vi "createOuterLoopClockIRQ.vi"(8 "error in (no error)":errorcluster, 11 "Boot in":refnum<class "Boot.lvclass">) -> (0 "error out":errorcluster, 2 "OuterLoopClockIRQ":refnum<class "IIRQ.lvclass">, 3 "Boot out":refnum<class "Boot.lvclass">)   [LabVIEW 2016, in "Boot.lvclass"]
uses:
  Boot.lvclass
  Common_RT_FPGA/IIRQ/IIRQ.lvclass
  Resources/OuterLoopClockIRQ/OuterLoopClockIRQ.lvclass
  D:/Code/ts_M1M3Support/Common_RT_FPGA/IIRQ/IIRQ.lvclass
  Boot.lvclass/Boot.ctl
  Resources/OuterLoopClockIRQ/OuterLoopClockIRQ.lvclass/OuterLoopClockIRQ.ctl
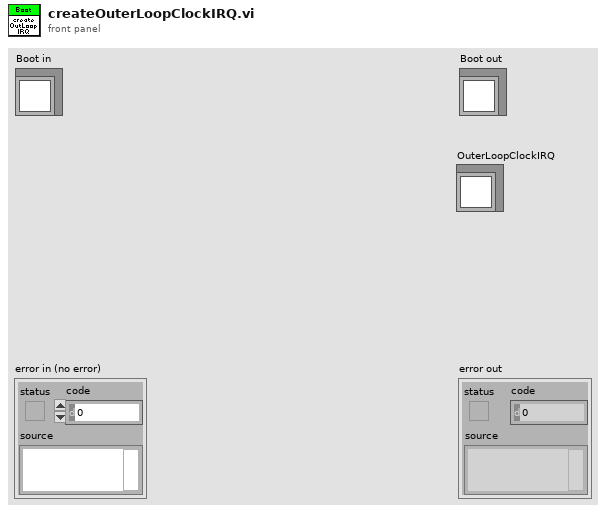
[diagram p1: front panel]
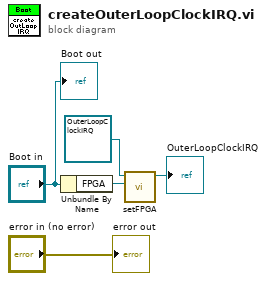
[diagram p0: block diagram]
diagram:
  n1 = Unbundle By Name("Boot in") -> ("FPGA"=w4:refnum<class "FPGA.lvclass">)
  n2 = call "setFPGA.vi"("FPGA"=w4, "OuterLoopClockIRQ in"=refnum<class "OuterLoopClockIRQ.lvclass"> refnum ("OuterLoopClockIRQ.lvclass")) -> ("OuterLoopClockIRQ out"=→"OuterLoopClockIRQ":refnum<class "OuterLoopClockIRQ.lvclass">)  [unwired: 9 in]
  "error out" <- "error in (no error)"
  "Boot out" <- "Boot in"
